vi "Open All Relays.vi"(8 "error in":errorcluster, 11 "2525 in":refnum<class "2525.lvclass">) -> (0 "error out":errorcluster, 3 "2525 out":refnum<class "2525.lvclass">)   [LabVIEW 2019, in "2525.lvlib" / "2525.lvclass"]
doc: "Open all relays is a static implementation because the state information in memory must be updated before opening the relays. This allows the end user to be aware of the switch state without requiring a query to the instrument."
uses:
  Library/2525.lvclass
  Library/2525.lvclass/2525.ctl
  builds/Instruments/SwitchMatrix.lvlibp/Library/SwitchMatrix.lvclass
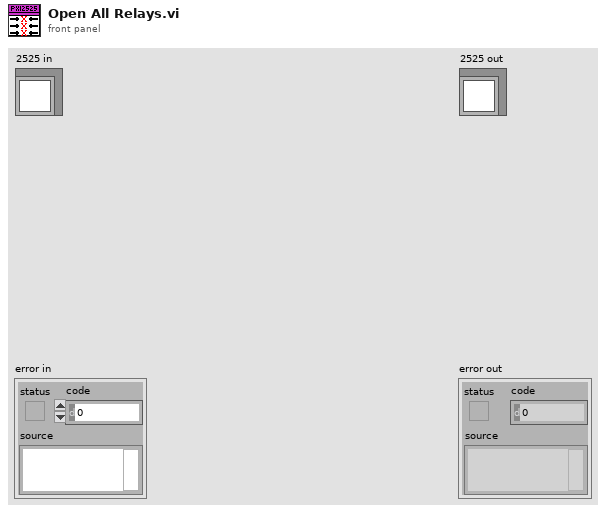
[diagram p1: front panel]
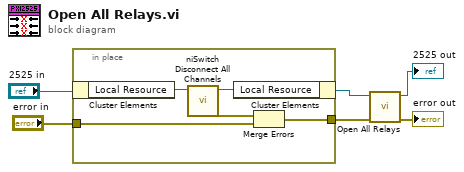
[diagram p0: block diagram]
diagram:
  n1 = in-place {
    in-place-border: "error in" -> [w8]
    in-place-border: [w7] -> w2
    n2 = in-place-cluster #1("2525 in") -> ("Local Resource"=w11:refnum<k15>)
    n3 = call <instrlib>:"niSwitch Disconnect All Channels.vi"("instrument handle"=w11) -> ("error out"=w9:errorcluster, "instrument handle out"=w10:refnum<k15>)  [unwired: 9 in]
    n4 = in-place-cluster #1("Local Resource"=w10) -> (w1:refnum<class "2525.lvclass">)
    n5 = Merge Errors(w9, w8) -> (w7:errorcluster)
  }
  n6 = call-parent "Open All Relays.vi"("error in"=w2, "SwitchMatrix in"=w1) -> ("error out"=→"error out":errorcluster, "SwitchMatrix out"=→"2525 out":refnum<class "2525.lvclass">)  [unwired: 8 in]
